vi "Frequency Demodulator.vi"(9 "Low cutoff freq: fl":dbl, 10 "Modulations\nFrequency":dbl, 11 "Waveform In":waveform(dbl)) -> (3 "Demodulated signal":waveform(dbl)(graph))   [LabVIEW 2014, in "Aquisicao de Dados.lvlib"]
uses:
  Aquisicao de Dados.lvlib
  <vilib>/Analysis/3filter.llb/Filter Passband Type.ctl
  <vilib>/Analysis/3filter.llb/Butterworth Filter (DBL).vi
  <vilib>/Analysis/NI_AALBase.lvlib
  <vilib>/Analysis/NI_AALPro.lvlib
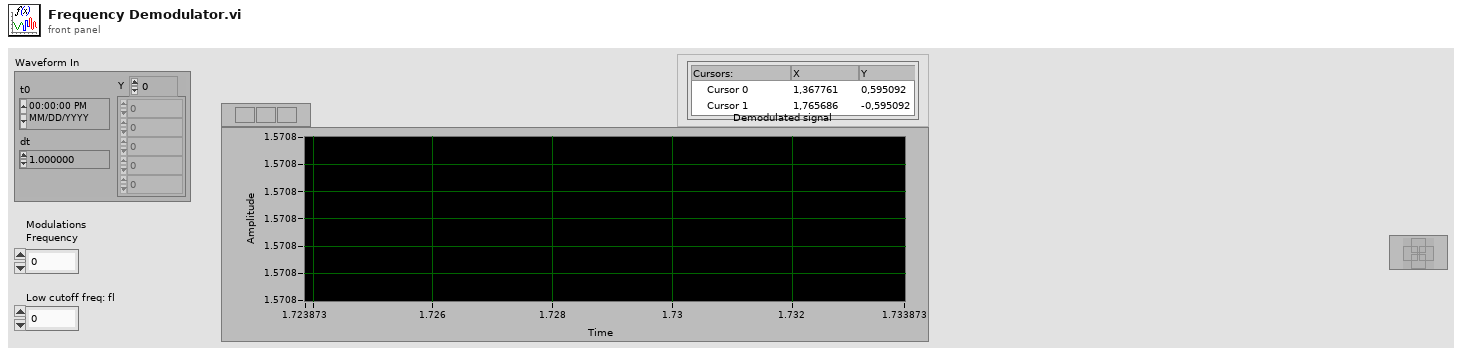
[diagram p1: front panel]
types:
  T1 = typedef "NI_AALBase.lvlib/Filter Passband Type.ctl" = enum32{"Lowpass", "Highpass", "Bandpass", "Bandstop"}
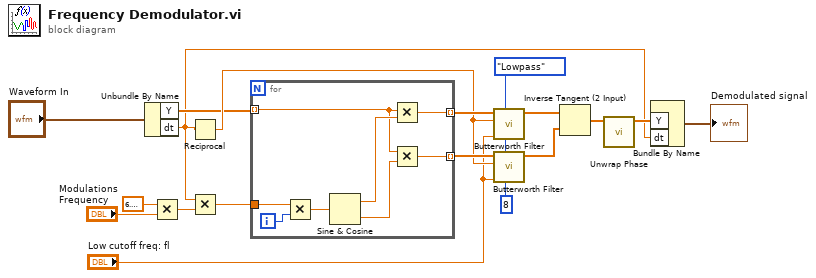
[diagram p0: block diagram]
diagram:
  w17 = Filter_Passband_Type."Lowpass" ("filter type")
  n1 = Unbundle By Name("Waveform In") -> ("Y"=w6:dbl[], "dt"=w1:dbl)
  n2 = Multiply(x=6.283185307179586, y="Modulations\nFrequency") -> (x*y=w5:dbl)
  n3 = Reciprocal(x=w1) -> (1/x=w8:dbl)
  n4 = Multiply(x=w1, y=w5) -> (x*y=w3:dbl)
  n5 = for {
    tunnel: w3 -> [w25]
    tunnel: w6 -> [w21] mode=indexing
    tunnel: [w20] -> w9 mode=indexing
    tunnel: [w19] -> w10 mode=indexing
    i -> [w26]
    n6 = Multiply(x=w25, y=w26) -> (x*y=w24:dbl)
    n7 = Sine & Cosine(0:w24) -> (1:w23:dbl, 2:w22:dbl)
    n8 = Multiply(x=w21, y=w23) -> (x*y=w20:dbl)
    n9 = Multiply(x=w21, y=w22) -> (x*y=w19:dbl)
  }
  n10 = call-poly <vilib>:"Butterworth Filter.vi"("filter type"=w17, "low cutoff freq: fl"="Low cutoff freq: fl", "sampling freq: fs"=w8, "X"=w9) -> ("Filtered X"=w11:dbl[])  [unwired: 4 in, 1 out]
  n11 = call-poly <vilib>:"Butterworth Filter.vi"("order"=8, "filter type"=w17, "low cutoff freq: fl"="Low cutoff freq: fl", "sampling freq: fs"=w8, "X"=w10) -> ("Filtered X"=w12:dbl[])  [unwired: 3 in, 1 out]
  n12 = Inverse Tangent (2 Input)(1:w12, 2:w11) -> (0:w13:dbl[])
  n13 = call <vilib>:"Unwrap Phase.vi"("Phase"=w13) -> ("Unwrapped Phase"=w14:dbl[])  [unwired: 9 in, 1 out]
  n14 = Bundle By Name("Y"=w14, "dt"=w1) -> (→"Demodulated signal":waveform(dbl))  [unwired: 1 in]
